vi "Read Voltage.vi"(8 "error in (no error)":errorcluster, 11 "PXIe-5172:Fetch Waveforms CFG in":refnum<class "Voltmeter CFG.lvclass">=refnum) -> (0 "error out":errorcluster, 2 "Voltage":dbl format="%#_g V", 3 "PXIe-5172:Fetch Waveforms CFG out":refnum<class "Voltmeter CFG.lvclass">)   [LabVIEW 2023, in "PXIe-5172.lvlib" / "Fetch Waveforms CFG.lvclass"]
uses:
  Fetch Waveforms CFG.lvclass
  <vilib>/Analysis/NI_AALBase.lvlib
  <vilib>/Analysis/baseanly.llb/Mean (DBL).vi
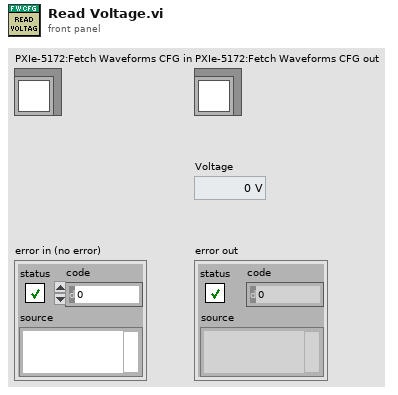
[diagram p1: front panel]
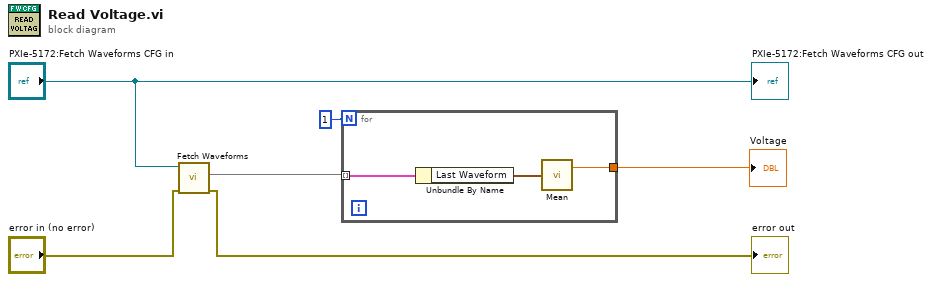
[diagram p0: block diagram]
diagram:
  n1 = call-dynamic "Fetch Waveforms.vi"("error in"="error in (no error)", "object in"="PXIe-5172:Fetch Waveforms CFG in") -> ("error out"=→"error out":errorcluster, "Last Waveforms"=w4:map{u8, waveform(dbl)})  [unwired: 7 in, 1 out]
  n2 = for {
    N: 1 -> [_]
    tunnel: [w9] -> w5
    tunnel: w4 -> [w8] mode=indexing
    n3 = Unbundle By Name(w8) -> ("Last Waveform"=w7:waveform(dbl))
    n4 = call-poly <vilib>:"Mean.vi"("X"=w7) -> ("mean"=w9:dbl)  [unwired: 1 out]
  }
  "Voltage" <- w5
  "PXIe-5172:Fetch Waveforms CFG out" <- "PXIe-5172:Fetch Waveforms CFG in"
